vi "_CSMOFGV Obtain.vi"(7 "Allowed Messages (Empty For All)":string[](array[string]), 8 "Error In":errorcluster caption="error in (no error)", 11 "Name (\"\" to Use UUID) In":string) -> (0 "error out":errorcluster, 1 "Create? (T)/Cached(F)":bool, 3 "CSM-Obj":T1={"info"={"Module Name"="", "Requested Name"="", "Group Name"="", "Mode"=enum."Stand Alone", "Allowed Messages"=[]}, "Refs"={"WatchDogQ"=refnum, "CSMDataDVR"=refnum, "Queue"={"HPriorityQ"=refnum, "LowPriorityQ"=refnum}, "GroupDataDVR"=refnum, "TagMap"=refnum, "ExitEvent"=refnum, "NewStateEvent"=refnum, "StatusEvent"=refnum, "InterruptEvent"=refnum}}, 4 "Name":string)   [LabVIEW 2017, in "Communicable State Machine.lvlib"]
uses:
  Communicable State Machine.lvlib
  _CSMObj.ctl
  _CSMObj-Info.ctl
  Typedef/_CSM_MODE.ctl
  _CSMObj-Refs.ctl
  _CSMObj-Data.ctl
  Priority Queue/Priority Queue.ctl
  Typedef/_Cross CSM State Data.ctl
  Typedef/_CSM_MSG_TYPE.ctl
  Typedef/_Cross CSM State Response.ctl
  Typedef/_CSM_Response Source Message.ctl
  Priority Queue/def-Data(LowPRI-Q).ctl
  _CSMObj-ModeData.ctl
  Typedef/_CSM Status Change Event Data.ctl
  _CSMOFGVOPER.ctl
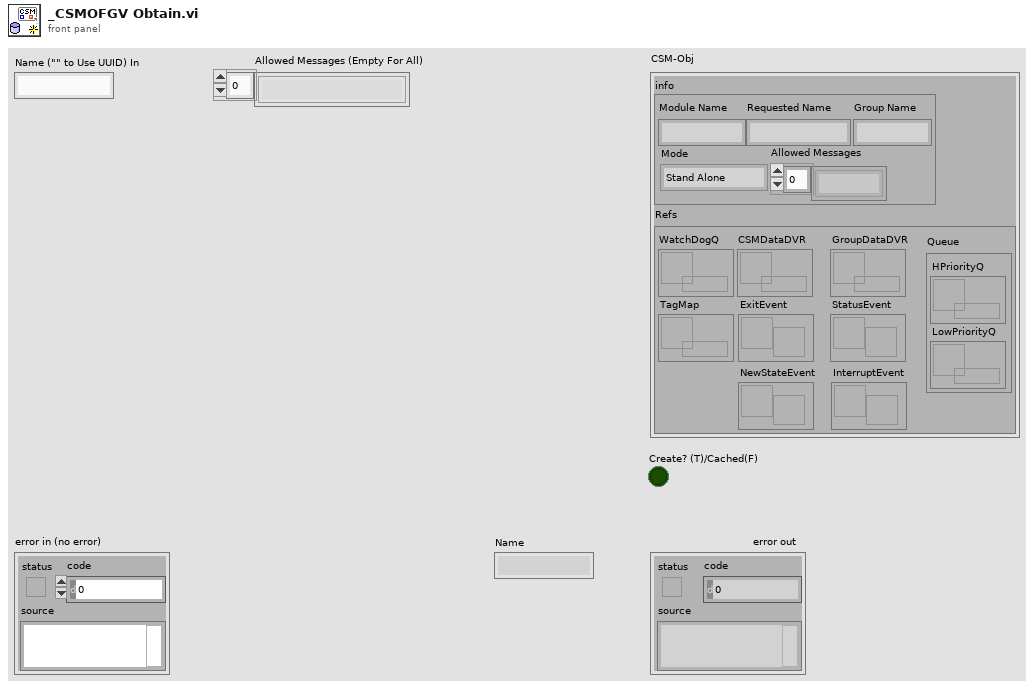
[diagram p1: front panel]
types:
  T1 = typedef "Communicable State Machine.lvlib/_CSMObj.ctl" = cluster{"info":T2, "Refs":T4}
  T2 = typedef "Communicable State Machine.lvlib/_CSMObj-Info.ctl" = cluster{"Module Name":string, "Requested Name":string, "Group Name":string, "Mode":T3, "Allowed Messages":string[]}
  T3 = typedef "Communicable State Machine.lvlib/_CSM_MODE.ctl" = enum16{"Not Exist", "Stand Alone", "CSM", "Worker", "Worker Agent", "Chain Node", "Chain"}
  T4 = typedef "Communicable State Machine.lvlib/_CSMObj-Refs.ctl" = cluster{"WatchDogQ":refnum<queue>, "CSMDataDVR":refnum<data-value>, "Queue":T5, "GroupDataDVR":refnum<data-value>, "TagMap":refnum<data-value>, "ExitEvent":refnum<user-event>, "NewStateEvent":refnum<user-event>, "StatusEvent":refnum<user-event>, "InterruptEvent":refnum<user-event>}
  T5 = typedef "Communicable State Machine.lvlib/Priority Queue.ctl" = cluster{"HPriorityQ":refnum<queue>, "LowPriorityQ":refnum<queue>}
  T6 = typedef "Communicable State Machine.lvlib/_CSMOFGVOPER.ctl" = enum16{"Create If not Exist", "Get By Name", "List", "Check If Name Exists", "Release", "Module Status", "Create Status Event Handler", "Destroy Status Event Handler", "Clear Invalid Objs"}
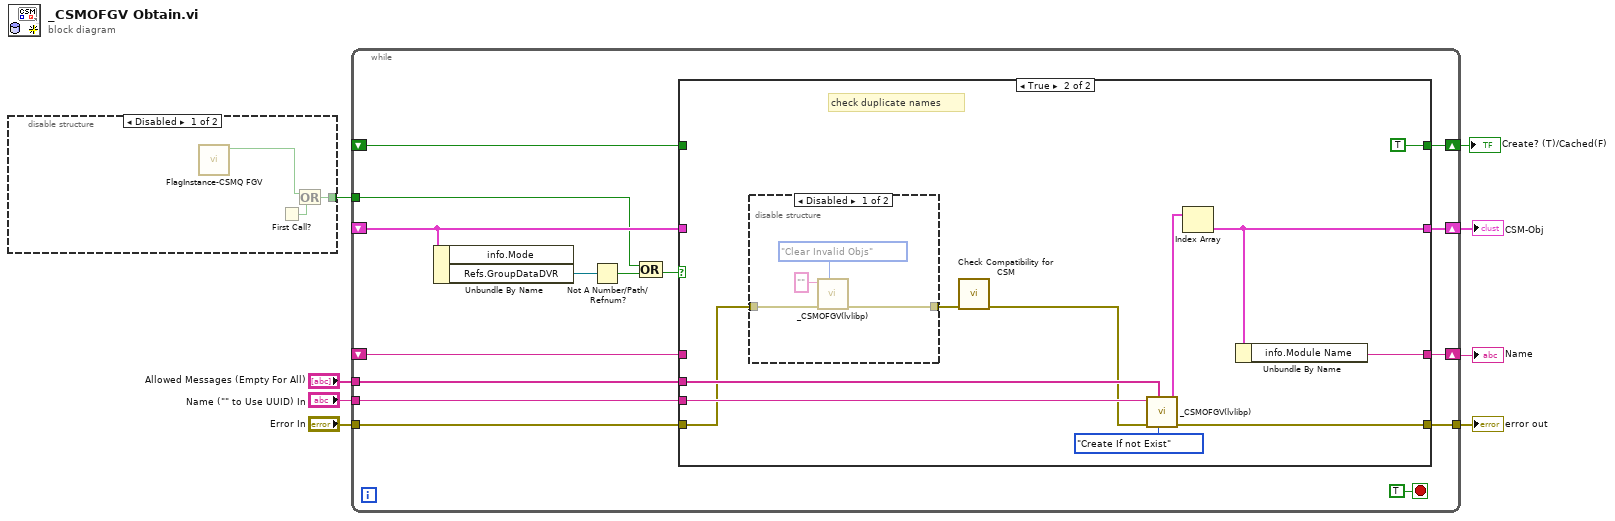
[diagram p0: block diagram]
diagram:
  n1 = disable-structure shown="Disabled" {
    disable-tunnel: [w11 _] -> w4
    frame Disabled {
      n2 = call "FlagInstance-CSMQ FGV.vi"() -> ("Changed"=w9:bool)  [unwired: 10 in, 1 out]
      n3 = First Call?() -> (First Call?: T/F=w10:bool)
      n4 = Or(x=w9, y=w10) -> (x .or. y?=w11:bool)
    }
    frame Enabled {
    }
  }
  n5 = while {
    shift-right: [w24] -> w5
    shift-left: _ -> [w19]
    tunnel: "Error In" -> [w23]
    tunnel: [w22] -> w7
    tunnel: "Name (\"\" to Use UUID) In" -> [w20]
    shift-right: [w17] -> w1
    shift-left: _ -> [w16]
    tunnel: w4 -> [w15]
    shift-right: [w13] -> w3
    shift-left: _ -> [w14]
    tunnel: "Allowed Messages (Empty For All)" -> [w12]
    stop <- TRUE stop-if-true
    n6 = Unbundle By Name(w19) -> ("Refs.GroupDataDVR"=w18:refnum<data-value>)  [unwired: 1 out]
    n7 = Not A Number/Path/Refnum?(number/path/refnum=w18) -> (NaN/Path/Refnum?=w25:bool)
    n8 = Compound Arithmetic op=OR(w15, w25) -> (w21:bool)
    n9 = case shown="True" w21 {
      tunnel: [w29 w35] -> w24
      tunnel: w19 -> [w29 _]
      tunnel: w23 -> [w28 w32]
      tunnel: [w28 w38] -> w22
      tunnel: w20 -> [_ w33]
      tunnel: [w27 w34] -> w17
      tunnel: w16 -> [w27 _]
      tunnel: w14 -> [_ _]
      tunnel: [_ TRUE] -> w13
      tunnel: w12 -> [_ w36]
      frame False {
      }
      frame True {
        # "check duplicate names"
        n10 = disable-structure shown="Disabled" {
          disable-tunnel: w32 -> [w43 w45]
          disable-tunnel: [w42 w45] -> w31
          frame Disabled {
            n11 = call "_CSMOFGV(lvlibp).vi"("Operation"=_CSMOFGVOPER."Clear Invalid Objs", "Error In"=w43, "Name (\"\" to Use UUID) In"="" ("Name (\"\" to Use UUID) in")) -> ("error out"=w42:errorcluster)  [unwired: 6 in, 2 out]
          }
          frame Enabled {
          }
        }
        n12 = call "Check Compatibility for CSM.vi"("Error in"=w31) -> ("Error out"=w30:errorcluster)  [unwired: 9 in, 1 out]
        n13 = call "_CSMOFGV(lvlibp).vi"("Operation"=_CSMOFGVOPER."Create If not Exist", "Allowed Messages (Empty For All)"=w36, "Error In"=w30, "Name (\"\" to Use UUID) In"=w33) -> ("error out"=w38:errorcluster, "Array"=w40:T1[])  [unwired: 5 in, 1 out]
        n14 = Index Array(array=w40) -> (element=w35:T1)  [unwired: 1 in]
        n15 = Unbundle By Name(w35) -> ("info.Module Name"=w34:string)
      }
    }
  }
  "error out" <- w7
  "CSM-Obj" <- w5
  "Name" <- w1
  "Create? (T)/Cached(F)" <- w3
